vi "Filter Sandbox.vi"() -> ()   [LabVIEW 2019]
doc: "This example demonstrates how a signal can be extracted from bandlimited noise using the filter VIs."
uses:
  <vilib>/Analysis/3filter.llb/Filter Passband Type.ctl
  <vilib>/Analysis/4window.llb/windowTd.ctl
  <vilib>/measure/maspectr.llb/Power Spectrum and PSD Export Mode.ctl
  <vilib>/Analysis/3filter.llb/IIR Cascade Filter with I.C. (DBL).vi
  <vilib>/Analysis/3filter.llb/IIR Filter with I.C. (DBL).vi
  <vilib>/addons/Digital Filter Design/Process.llb/DFD Filtering with State (Wfm).vi
  <vilib>/Analysis/3filter.llb/Butterworth Filter (DBL).vi
  <vilib>/addons/Digital Filter Design/Process.llb/DFD Filtering (Wfm NChan).vi
  <vilib>/measure/maspectr.llb/FFT Power Spectrum and PSD for N Chan.vi
  <vilib>/Analysis/NI_AALBase.lvlib
  <vilib>/addons/Digital Filter Design/NI_DigFilterLicensed.lvlib
  <vilib>/measure/NI_MABase.lvlib
  DSP.lvclass
  <vilib>/measure/NI_MAPro.lvlib
  <vilib>/Analysis/NI_AALPro.lvlib
panel:
  in  "Sine Amplitude (V)":dbl(slide)=10.0 scale=0.0..200.0
  in  "harmonics":i32
  out "PS Waveform":cluster{"f0":dbl, "df":dbl, "magnitude":dbl[]}[](graph)
  in  "Q":dbl
  in  "notch (Hz)":dbl
  out "Numeric":i32
  out "Waveform Graph 2":waveform(dbl)[](graph)
  in  "Sample rate (Hz)":dbl=1000.0
  in  "Stop":bool
  in  "Filter Order":i32(slide)=5 scale=0.0..10.0
  in  "Cut-Off Frequency (Hz)":dbl(slide)=20.0 scale=0.0..100.0
  in  "Sine Frequency (Hz)":dbl(slide)=10.0 scale=0.0..200.0
  # "Notch Filter:"
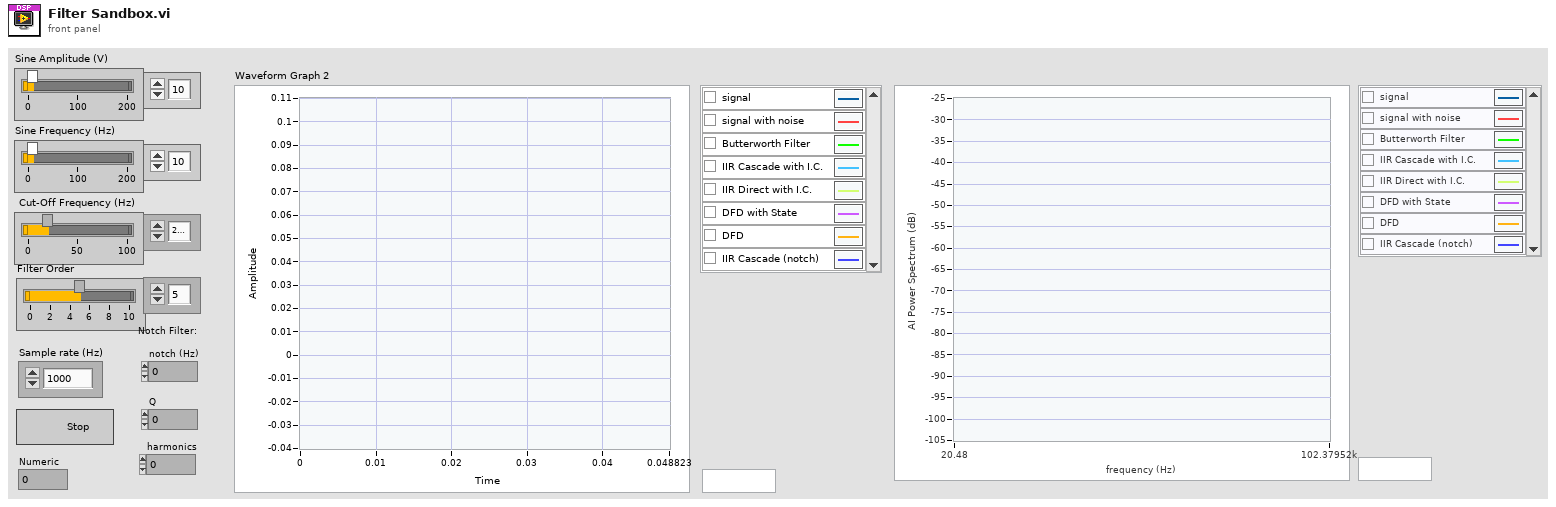
[diagram p1: front panel]
types:
  T1 = cluster{"averaging mode":enum16{"No averaging", "Vector averaging", "RMS averaging", "Peak hold"}, "weighting mode":enum16{"Linear", "Exponential"}, "number of averages":u32}
  T2 = enum16{"Sine Wave", "Triangle Wave", "Square Wave", "Sawtooth Wave"}
  T3 = typedef "NI_MAPro.lvlib/Power Spectrum and PSD Export Mode.ctl" = u16
  T4 = typedef "NI_AALPro.lvlib/windowTd.ctl" = u32
  T5 = typedef "NI_AALBase.lvlib/Filter Passband Type.ctl" = enum32{"Lowpass", "Highpass", "Bandpass", "Bandstop"}
  T6 = cluster{"filter structure":enum32{"IIR 2nd Order", "IIR 4th Order"}, "Reverse Coefficients":dbl[], "Forward Coefficients":dbl[]}
  T7 = typedef "NI_DigFilterLicensed.lvlib/DFD Filter Obj.ctl" = cluster{"mSRate_Fs":dbl, "mSRate_Version":string, "mSRate_Comments":string, "mSRate_OrgCoef":T8, "mSRate_CurCoef":T8, "mSRate_Quantized?":bool, "mSRate_QCoef":T8, "mSRate_QSettings":T10[], "mSRate_Order":i32, "mSRate_Scaling":cluster{"mSRate_ScaleByPowerOf2?":bool, "mSRate_ScaleType":T12}}
  T8 = typedef "NI_DigFilterLicensed.lvlib/DFD Filter Coef.ctl" = cluster{"type":T9, "gain":dbl, "coef a (k)":dbl[], "coef b (v)":dbl[]}
  T9 = typedef "NI_DigFilterLicensed.lvlib/DFD Filter Structure Type Selector.ctl" = enum16{"Undefined", "FIR Direct Form", "FIR Direct Form Transposed", "FIR Symmetric", "FIR Antisymmetric", "IIR Direct Form I", "IIR Direct Form I Transposed", "IIR Direct Form II", "IIR Direct Form II Transposed", "IIR Cascaded Second Order Sections Form I", "IIR Cascaded Second Order Sections Form I Transposed", "IIR Cascaded Second Order Sections Form II", "IIR Cascaded Second Order Sections Form II Transposed", "Lattice Allpass (basic sections)", "Lattice Allpass (one multiplier sections)", "Lattice Allpass (normalized sections)", "Lattice AR (basic sections)", "Lattice AR (one multiplier sections)", "Lattice AR (normalized sections)", "Lattice MA (minimum phase)", "Lattice MA (maximum phase)", "Lattice ARMA (basic sections)", "Lattice ARMA (one multiplier sections)", "Lattice ARMA (normalized sections)"}
  T10 = typedef "NI_DigFilterLicensed.lvlib/dfd_Internal Quantization Settings.ctl" = cluster{"source":T11, "wl":i16, "iwl":i16, "overflow mode":enum16{"Saturation", "Wrap"}, "rounding mode":enum16{"Nearest", "Truncation"}, "signed?":bool}
  T11 = typedef "NI_DigFilterLicensed.lvlib/dfd_Internal Quantization Srcs.ctl" = u16
  T12 = typedef "NI_DigFilterLicensed.lvlib/DFD Coef Norm Type.ctl" = enum16{"No Norm", "Time Domain 1-Norm", "Time Domain 2-Norm", "Time Domain Inf-Norm"}
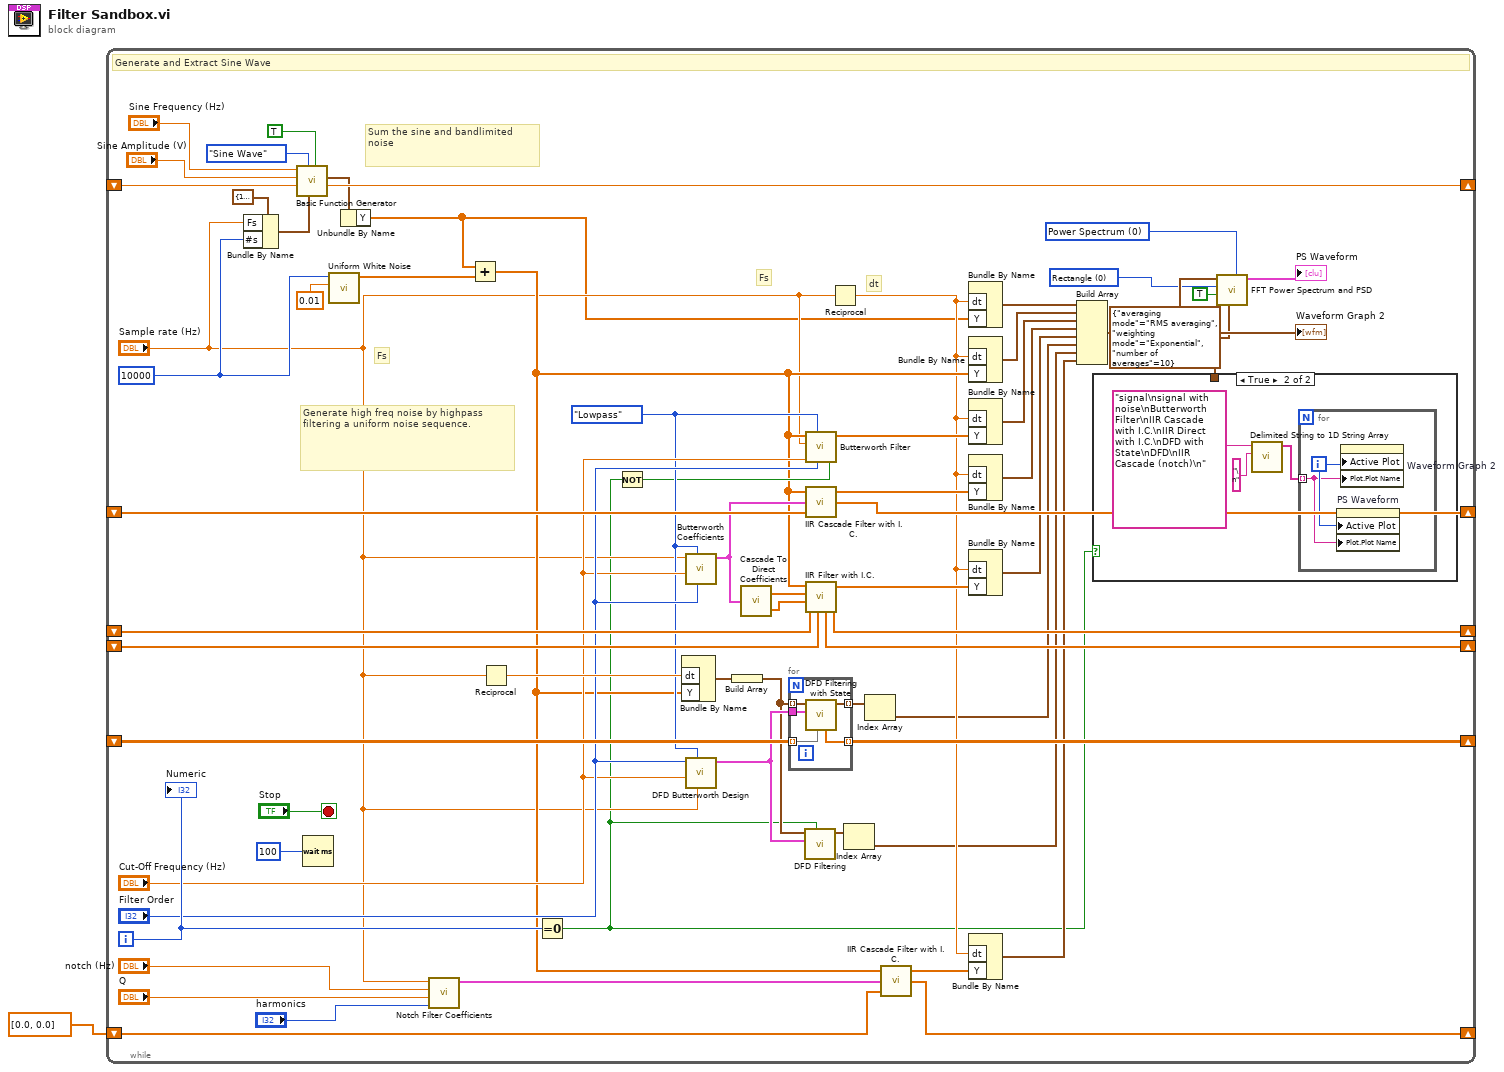
[diagram p0: block diagram]
diagram:
  n1 = while {
    shift-right: [w56] -> _
    shift-left: _ -> [w63]
    shift-right: [w58] -> _
    shift-left: _ -> [w57]
    shift-right: [w52] -> _
    shift-left: _ -> [w50]
    shift-right: [w51] -> _
    shift-left: _ -> [w49]
    shift-right: [w30] -> _
    shift-left: dbl[] [0.0, 0.0] ("Final X Conditions") -> [w23]
    shift-right: [w36] -> _
    shift-left: _ -> [w35]
    i -> [w62]
    stop <- "Stop" stop-if-true
    w3 = T3 0 items=["Power Spectrum", "Power Spectral Density"] ("export mode")
    w4 = T4 0 items=["Rectangle"=0, "Hanning"=1, "Hamming"=2, "Blackman-Harris"=3, "Exact Blackman"=4, "Blackman"=5, "Flat Top"=6, "4 Term B-Harris "=7, "7 Term B-Harris"=8, "Low Sidelobe"=9, "Blackman Nuttall"=11, "Triangle"=30, "Bartlett-Hanning"=31, "Bohman"=32, "Parzen"=33, "Welch"=34, "Kaiser"=60, "Dolph-Chebyshev"=61, "Gaussian"=62] ("window")
    w41 = Filter_Passband_Type."Lowpass" ("filter type")
    w21 = 10000
    # "Fs"
    # "dt"
    # "Fs"
    # "Sum the sine and bandlimited noise"
    # "Generate high freq noise by highpass filtering a uniform noise sequence."
    # "Generate and Extract Sine Wave"
    n2 = Bundle By Name(cluster=cluster{"Fs":dbl, "#s":dbl} {"Fs"=1000.0, "#s"=1000.0} ("sampling info"), "Fs"="Sample rate (Hz)", "#s"=w21) -> (w33:cluster{"Fs":dbl, "#s":dbl})
    n3 = call <vilib>:"Basic Function Generator.vi"("reset signal"=TRUE, "sampling info"=w33, "signal type"=T2."Sine Wave", "phase"=w35, "amplitude"="Sine Amplitude (V)", "frequency"="Sine Frequency (Hz)") -> ("phase out"=w36:dbl, "signal out"=w31:waveform(dbl))  [unwired: 3 in, 1 out]
    n4 = Wait (ms)(milliseconds to wait=u32 100) -> ()  [unwired: 1 out]
    n5 = call <vilib>:"Uniform White Noise.vi"("amplitude"=0.01, "samples"=w21) -> ("uniform white noise"=w6:dbl[])  [unwired: 8 in, 1 out]
    n6 = Unbundle By Name(w31) -> ("Y"=w13:dbl[])
    n7 = call "Notch Filter Coefficients.vi"("harmonics"="harmonics", "Q"="Q", "notch (Hz)"="notch (Hz)", "Sample rate (Hz)"="Sample rate (Hz)") -> ("IIR Filter Cluster"=w24:T6)  [unwired: 5 in, 2 out]
    n8 = Add(x=w13, y=w6) -> (x+y=w17:dbl[])
    n9 = Reciprocal(x="Sample rate (Hz)") -> (1/x=w48:dbl)
    n10 = Equal To 0?(x=w62) -> (x = 0?=w12:bool)
    n11 = Not(x=w12) -> (.not. x?=w40:bool)
    n12 = Bundle By Name("dt"=w48, "Y"=w17) -> (w26:waveform(dbl))  [unwired: 1 in]
    n13 = call <vilib>:"Butterworth Coefficients.vi"("order"="Filter Order", "filter type"=w41, "low cutoff freq: fl"="Cut-Off Frequency (Hz)", "sampling freq: fs"="Sample rate (Hz)") -> ("IIR Filter Cluster"=w29:T6)  [unwired: 6 in, 1 out]
    n14 = call <vilib>:"DFD Butterworth Design.vi"("fs [Hz]"="Sample rate (Hz)", "filter type"=w41, "low cutoff freq [Hz]"="Cut-Off Frequency (Hz)", "order"="Filter Order") -> ("filter out"=w47:T7)  [unwired: 6 in, 1 out]
    n15 = Build Array(w26) -> (w25:waveform(dbl)[])
    n16 = call <vilib>:"Cascade To Direct Coefficients.vi"("IIR Filter Cluster"=w29) -> ("Reverse Coefficients"=w54:dbl[], "Forward Coefficients"=w53:dbl[])
    n17 = for {
      tunnel: [w76] -> w58 mode=indexing
      tunnel: w57 -> [w75] mode=indexing
      tunnel: w47 -> [w74]
      tunnel: w25 -> [w73] mode=indexing
      tunnel: [w72] -> w44 mode=indexing
      n18 = call-poly <vilib>:"DFD Filtering with State.vi"("state in"=w75, "filter"=w74, "signal in"=w73) -> ("signal out"=w72:waveform(dbl), "state out"=w76:dbl[])  [unwired: 6 in, 1 out]
    }
    n19 = call-poly <vilib>:"DFD Filtering.vi"("init? (F)"=w12, "filter"=w47, "signal in"=w25) -> ("signal out"=w45:waveform(dbl)[])  [unwired: 7 in, 1 out]
    n20 = call-poly <vilib>:"Butterworth Filter.vi"("init/cont (init:F)"=w40, "order"="Filter Order", "filter type"=w41, "low cutoff freq: fl"="Cut-Off Frequency (Hz)", "sampling freq: fs"="Sample rate (Hz)", "X"=w17) -> ("Filtered X"=w60:dbl[])  [unwired: 2 in, 1 out]
    n21 = call-poly <vilib>:"IIR Cascade Filter with I.C..vi"("Initial Filter State"=w63, "IIR Filter Cluster"=w29, "X"=w17) -> ("Final Filter State"=w56:dbl[], "Filtered X"=w61:dbl[])  [unwired: 1 out]
    n22 = call-poly <vilib>:"IIR Filter with I.C..vi"("Initial Y Conditions"=w49, "Initial X Conditions"=w50, "Forward Coefficients"=w53, "Reverse Coefficients"=w54, "X"=w17) -> ("Final X Conditions"=w52:dbl[], "Final Y Conditions"=w51:dbl[], "Filtered X"=w55:dbl[])  [unwired: 2 in, 1 out]
    n23 = Reciprocal(x="Sample rate (Hz)") -> (1/x=w15:dbl)
    n24 = Index Array(array=w45) -> (element=w11:waveform(dbl))  [unwired: 1 in]
    n25 = Index Array(array=w44) -> (element=w10:waveform(dbl))  [unwired: 1 in]
    n26 = call-poly <vilib>:"IIR Cascade Filter with I.C..vi"("Initial Filter State"=w23, "IIR Filter Cluster"=w24, "X"=w17) -> ("Final Filter State"=w30:dbl[], "Filtered X"=w39:dbl[])  [unwired: 1 out]
    n27 = Bundle By Name("dt"=w15, "Y"=w13) -> (w43:waveform(dbl))  [unwired: 1 in]
    n28 = Bundle By Name("dt"=w15, "Y"=w17) -> (w18:waveform(dbl))  [unwired: 1 in]
    n29 = Bundle By Name("dt"=w15, "Y"=w60) -> (w65:waveform(dbl))  [unwired: 1 in]
    n30 = Bundle By Name("dt"=w15, "Y"=w61) -> (w59:waveform(dbl))  [unwired: 1 in]
    n31 = Bundle By Name("dt"=w15, "Y"=w55) -> (w16:waveform(dbl))  [unwired: 1 in]
    n32 = Bundle By Name("dt"=w15, "Y"=w39) -> (w38:waveform(dbl))  [unwired: 1 in]
    n33 = Build Array(w43, w18, w65, w59, w16, w10, w11, w38) -> (w9:waveform(dbl)[])
    "Waveform Graph 2" <- w9
    n34 = case shown="True" w12 {
      tunnel: w9 -> [_ _]
      frame False {
      }
      frame True {
        n35 = call <vilib>:"Delimited String to 1D String Array.vi"("delimiter"="\n", "delimited string"="signal\nsignal with noise\nButterworth Filter\nIIR Cascade with I.C.\nIIR Direct with I.C.\nDFD with State\nDFD\nIIR Cascade (notch)\n" ("String")) -> ("string array"=w69:string[])  [unwired: 9 in]
        n36 = for {
          tunnel: w69 -> [w70] mode=indexing
          i -> [w71]
          n37 = property on="PS Waveform" class="WFGraph (strict)"("Active Plot"=w71, "Plot.Plot Name"=w70) -> ()  [unwired: 2 in, 2 out]
          n38 = property on="Waveform Graph 2" class="WFGraph (strict)"("Active Plot"=w71, "Plot.Plot Name"=w70) -> ()  [unwired: 2 in, 2 out]
        }
      }
    }
    n39 = call-poly <vilib>:"FFT Power Spectrum and PSD.vi"("export mode"=w3, "averaging parameters"=T1 {"averaging mode"=enum."RMS averaging", "weighting mode"=enum."Exponential", "number of averages"=10}, "dB On (F)"=TRUE, "window"=w4, "time signals"=w9) -> ("Power Spectrum / PSD"=→"PS Waveform":cluster{"f0":dbl, "df":dbl, "magnitude":dbl[]}[])  [unwired: 3 in, 3 out]
    "Numeric" <- w62
  }
